vi "UDP Receiver.vi"() -> ()   [LabVIEW 2013]
panel:
  out "Buffer In":u8[](array[numeric])=[204, 0, 0, 0, 0, 0, 0, 0, 0, 0, 0, 0, 0, 0, 0, 0, 0, 0, 0, 0, 0, 0, 0, 0, 0, 0, 0, 0, 0, 0, 0, 0, 85, 170] format="0x%x"
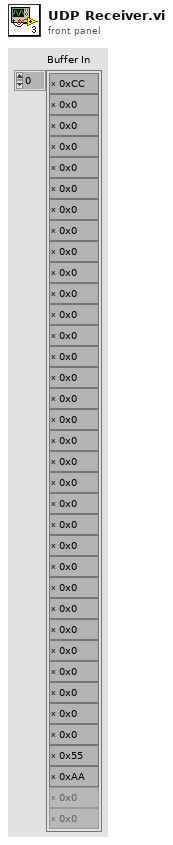
[diagram p1: front panel]
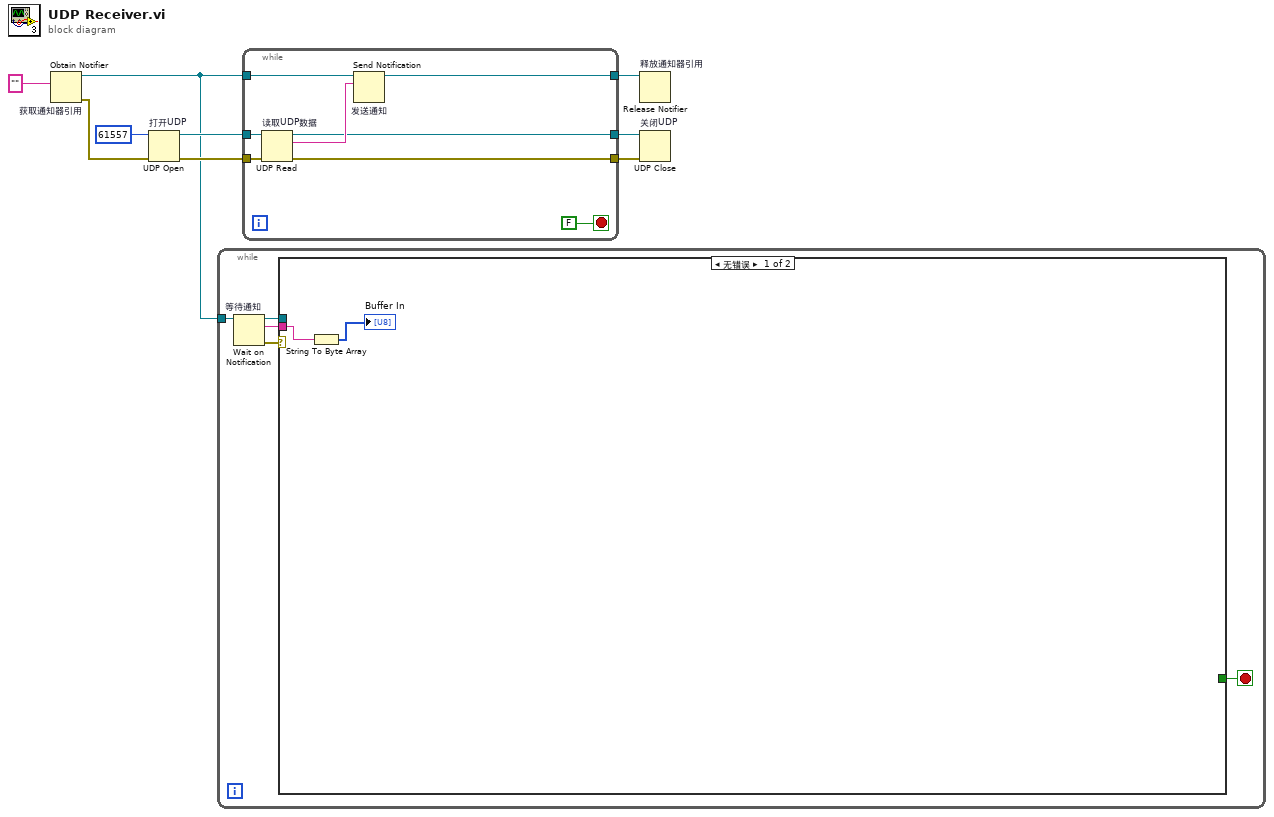
[diagram p0: block diagram]
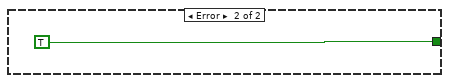
[diagram p2: hidden frame]
diagram:
  n1 = Obtain Notifier "获取通知器引用"(notification data type="" ("data out")) -> (notifier out=w1:refnum<notifier>, error out=w6:errorcluster)  [unwired: 3 in, 1 out]
  n2 = UDP Open "打开UDP"(8:w6, 11:u16 61557 ("port")) -> (port=w7:refnum<k16>, 0:w5:errorcluster)  [unwired: 3 in, 1 out]
  n3 = while {
    tunnel: w1 -> [w14]
    stop <- w10 stop-if-true
    n4 = Wait on Notification "等待通知"(notifier=w14) -> (notifier out=w12:refnum<notifier>, notification=w13:string, error out=w11:errorcluster)  [unwired: 3 in, 1 out]
    n5 = case shown="无错误" w11 {
      tunnel: w13 -> [w16 _]
      tunnel: w12 -> [_ _]
      tunnel: [_ TRUE] -> w10
      frame No Error {
        n6 = String To Byte Array(string=w16) -> (unsigned byte array=→"Buffer In":u8[])
      }
      frame Error {
      }
    }
  }
  n7 = while {
    tunnel: w1 -> [w25]
    tunnel: w7 -> [w23]
    tunnel: w5 -> [w22]
    tunnel: [w21] -> w4
    tunnel: [w20] -> w3
    tunnel: [w19] -> w2
    stop <- FALSE stop-if-true
    n8 = UDP Read "读取UDP数据"(connection ID=w23, 8:w22) -> (data out=w24:string, error out=w19:errorcluster, 3:w20:refnum<k16>)  [unwired: 2 in, 2 out]
    n9 = Send Notification "发送通知"(notification=w24, notifier=w25) -> (notifier out=w21:refnum<notifier>)  [unwired: 1 in, 1 out]
  }
  n10 = Release Notifier "释放通知器引用"(notifier=w4) -> ()  [unwired: 2 in, 3 out]
  n11 = UDP Close "关闭UDP"(connection ID=w3, 8:w2) -> ()  [unwired: 2 out]
